vi "FPGA 796xR - Backup20170922A.vi"() -> ()   [LabVIEW 2015]
uses:
  Controls/FPGA_Frame State.ctl
  <vilib>/Platform/TimedLoop/XDataNode/timing_clust.ctl
  <vilib>/Platform/TimedLoop/XDataNode/nitl_modes.ctl
  <vilib>/Platform/TimedLoop/XDataNode/wakeup.ctl
  <vilib>/rvi/Emulation/niFpgaSctlEmulationGetInTimedLoop.vi
  <vilib>/rvi/Emulation/niFpgaProcessEmulError.vi
  <vilib>/rvi/Emulation/niFpgaEmulationReportErrorSimple.vi
  <vilib>/rvi/Emulation/niFpgaGetClockAttributes.vi
  <vilib>/rvi/Emulation/niFpgaCriticalErrorInLSC.vi
  <vilib>/rvi/eio/common/nirviEmuTemplateMethod_errors.vi
  <vilib>/rvi/Memory/Memory_Emulation/nirvimemoryFastEmulation.vi
  <vilib>/rvi/Memory/Memory_Emulation/nirvimemoryEmulation.vi
  <vilib>/rvi/Emulation/niFpgaEmulationIsFPGAContextNoSignature.vi
  <vilib>/rvi/DataTransferAndStorage/Container/Common/niFpgaContainerGetUniqueNameForEmu.vi
  <vilib>/rvi/errors/nirviReportUnexpectedCaseInternalError (U32).vi
  <vilib>/rvi/interface/RandomDataEmulation/niFpgaRandomDataHandleErrors.vi
  <vilib>/Platform/TimedLoop/XDataNode/XDataNode.xnode
  <vilib>/eio/EIONode/EIONode.xnode
  <vilib>/rvi/DataTransferAndStorage/Container/XNode/niFpgaContainer.xnode
  <vilib>/rvi/FXPMathLib/FxpMul/XNode/nifxpmath_Multiplier.xnode
  <vilib>/rvi/FXPMathLib/FxpAdd/XNode/nifxpmath_Add.xnode
  <vilib>/rvi/interface/RandomDataEmulation/nirviRandomDataFpgaReadWriteTemplate.vi
  <vilib>/Platform/TimedLoop/XDataNode/XDNodeRunTimeDep.lvlib
  <instrlib>/_niInstr/Basic Elements/v1/FPGA/niInstr Basic Elements v1 FPGA.lvlib
  <vilib>/rvi/FXPMathLib/sim/FxpSim.dll
panel:
  in  "Divide":u8
  out "Acq. Point Dis.":u16
  in  "Acq.Start":u16
  in  "Acq.Start FXP":fxp<+,18,0>
  out "Acq Pixel Number":u32
  out "AcqPoint 元素数量":u32
  in  "Microscope":enum16{"Miniature", "Benchtop"}(ring)
  in  "FOCUS":bool
  out "Wait Frame State":T1
  in  "Line":u16
  in  "Pixel/Line":u16
  out "Adapter Module Present":bool
  out "Adapter Module ID Expected":u32
  out "Adapter Module ID Inserted":u32
  out "Adapter Module Initialization Done":bool
  out "Adapter Module ID Mismatch":bool
  in  "Adapter Module Do User Command Commit":bool caption="(Mech Action: Latch)"
  in  "Adapter Module User Command":u8
  out "Adapter Module User Command Idle":bool
  out "Adapter Module User Command Status":u8
  in  "Adapter Module User Data 0":u8
  in  "Adapter Module User Data 1":u8
  out "Adapter Module PLL Locked":bool
  # "Acquisition Parameters"
  # "Acquisition Control"
  # "User Command Load"
  # "Fpga status"
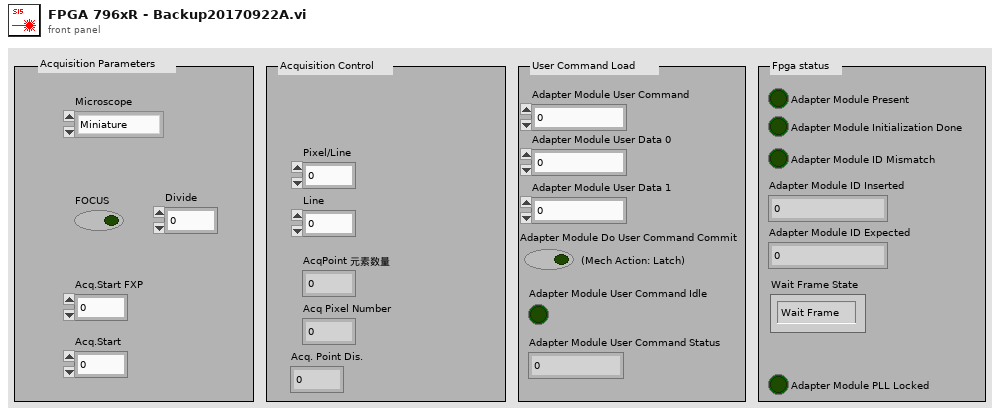
[diagram p1: front panel]
types:
  T1 = typedef "FPGA_Frame State.ctl" = enum16{"Wait Frame", "Start Frame", "Framing"}
  T2 = typedef "XDNodeRunTimeDep.lvlib/timing_clust.ctl" = cluster{"Expected End [f-1]":u64, "Actual End [f-1]":u64, "Finished Late? [f-1]":bool, "Expected End [i-1]":u64, "Actual End [i-1]":u64, "Finished Late? [i-1]":bool, "Expected Start [i]":u64, "Actual Start [i]":u64, "Expected Start [f]":u64, "Actual Start [f]":u64, "Source Name":string, "Structure Name":string, "Period":i64, "Deadline":i64, "Offset":i64, "Start":i64, "Priority":i32, "Timeout":i32, "Mode":T3, "Wakeup Reason":T4, "Error":errorcluster, "Source Type":string, "Secondary Source Type":string, "Global End Time":u64, "Global Start Time":u64, "Frame Duration":u64, "Iteration Duration":u64, "Assigned CPU":i32, "I/O Scan Engine Mode":u32}
  T3 = typedef "XDNodeRunTimeDep.lvlib/nitl_modes.ctl" = enum32{"No Change", "Process missed periods, maintain original phase", "Discard missed periods, maintain original phase", "Process missed periods, ignore original phase", "Discard missed periods, ignore original phase"}
  T4 = typedef "XDNodeRunTimeDep.lvlib/wakeup.ctl" = enum32{"Normal", "Aborted", "Asynchronous wakeup", "Timing source error", "Timed loop error", "Timeout"}
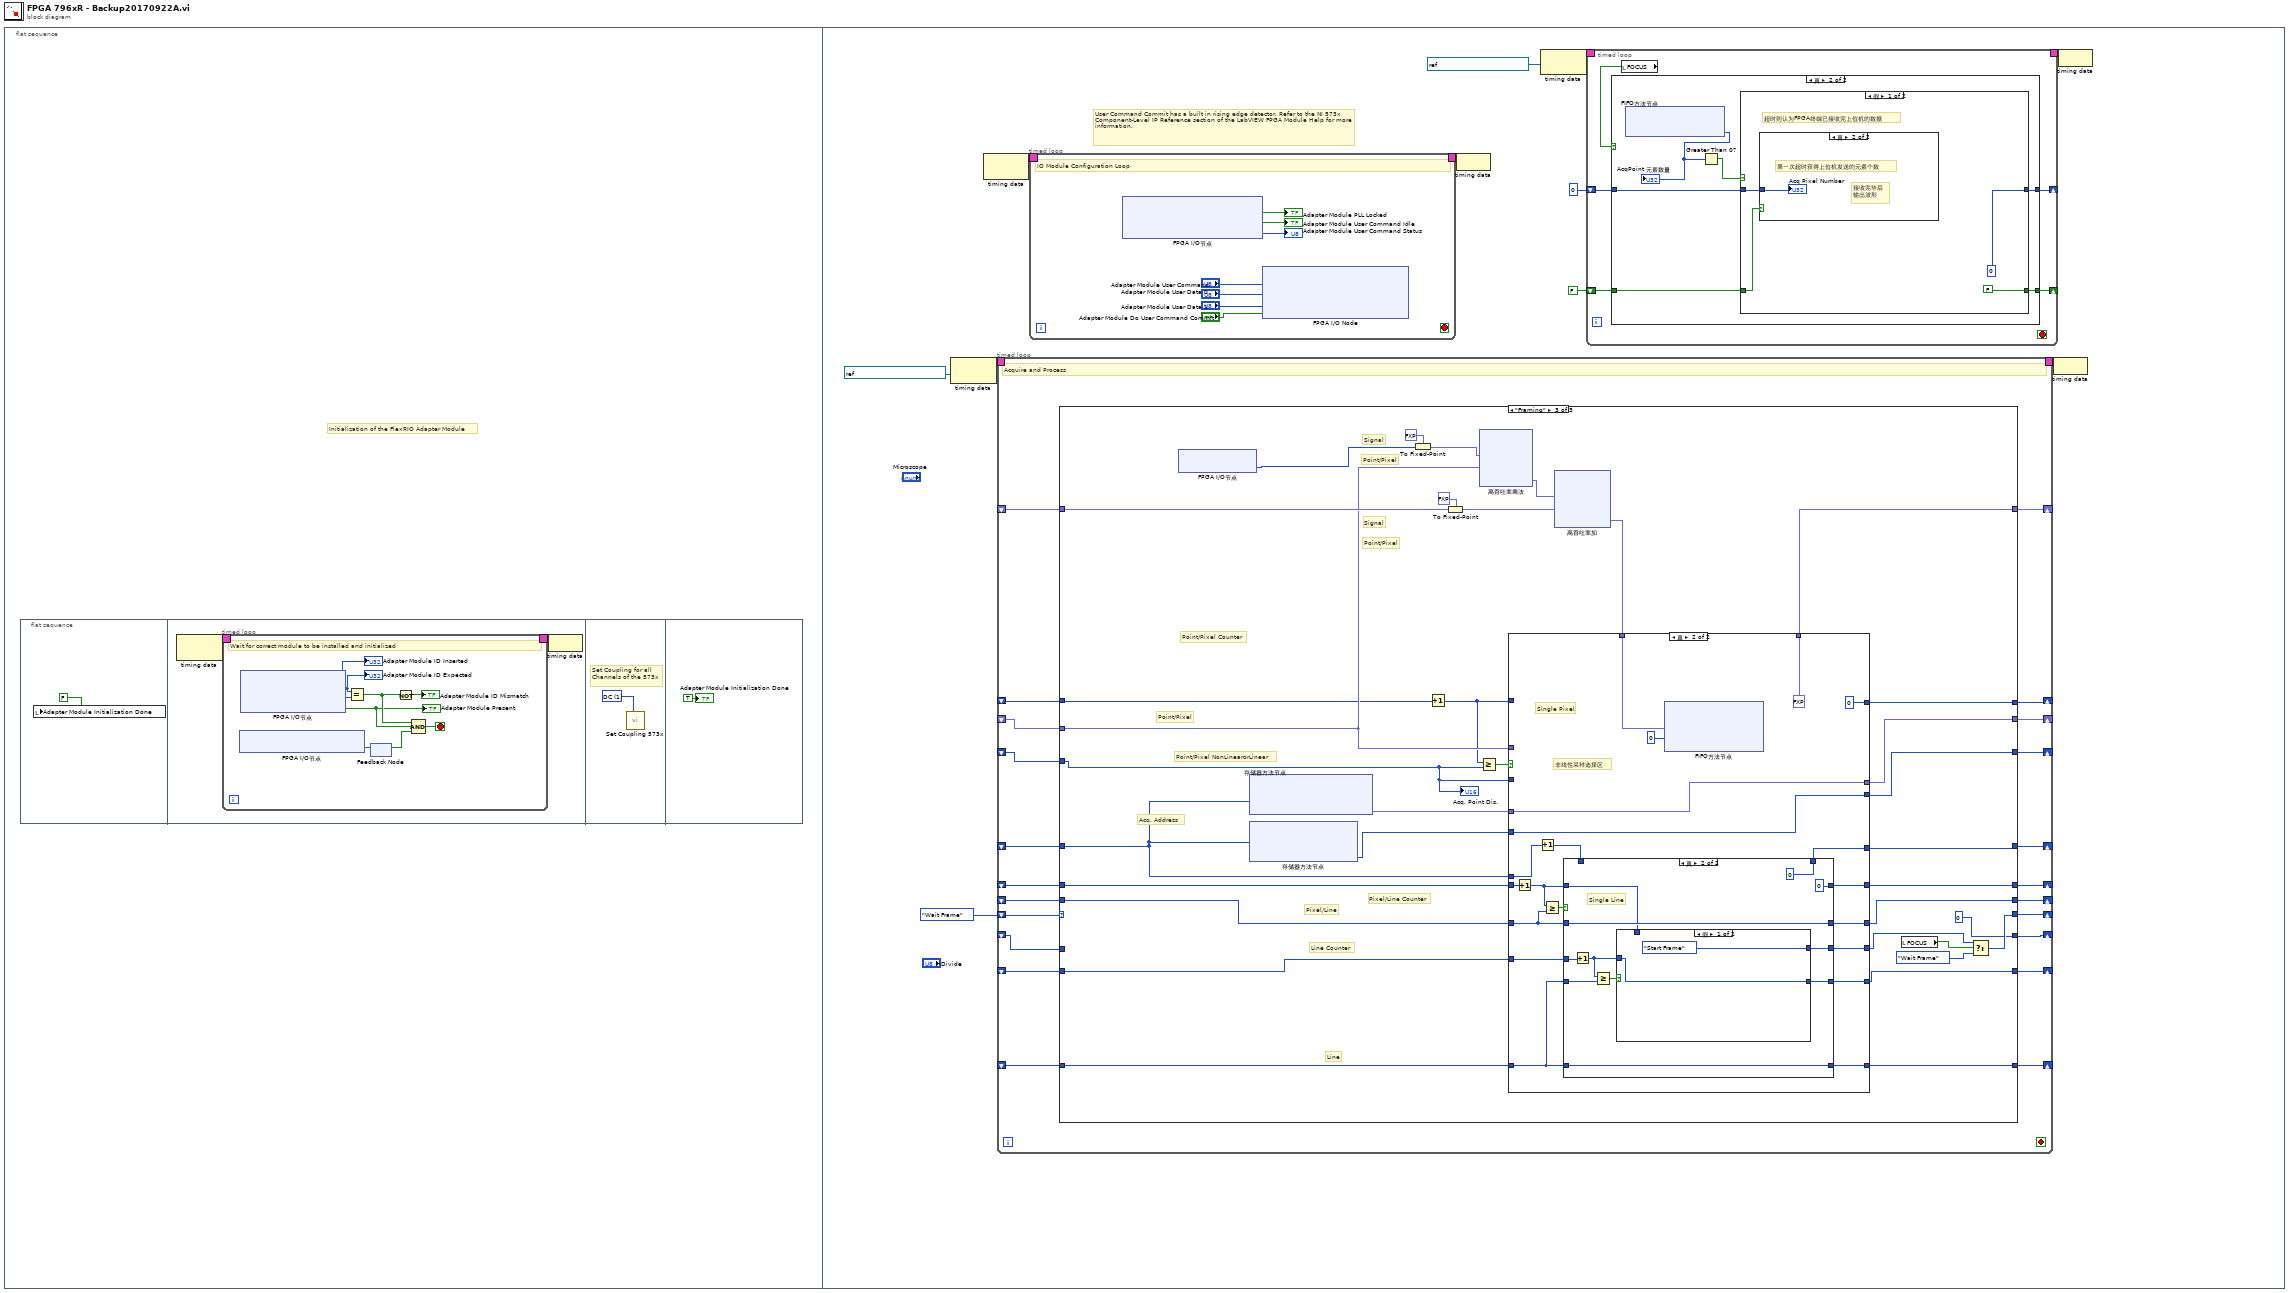
[diagram p0: block diagram]
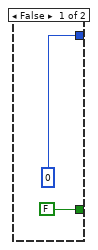
[diagram p2: hidden frame]
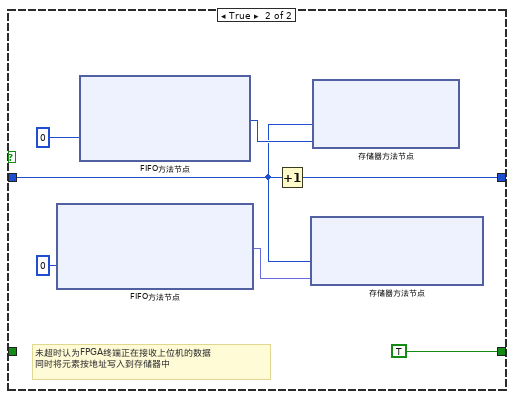
[diagram p4: hidden frame]
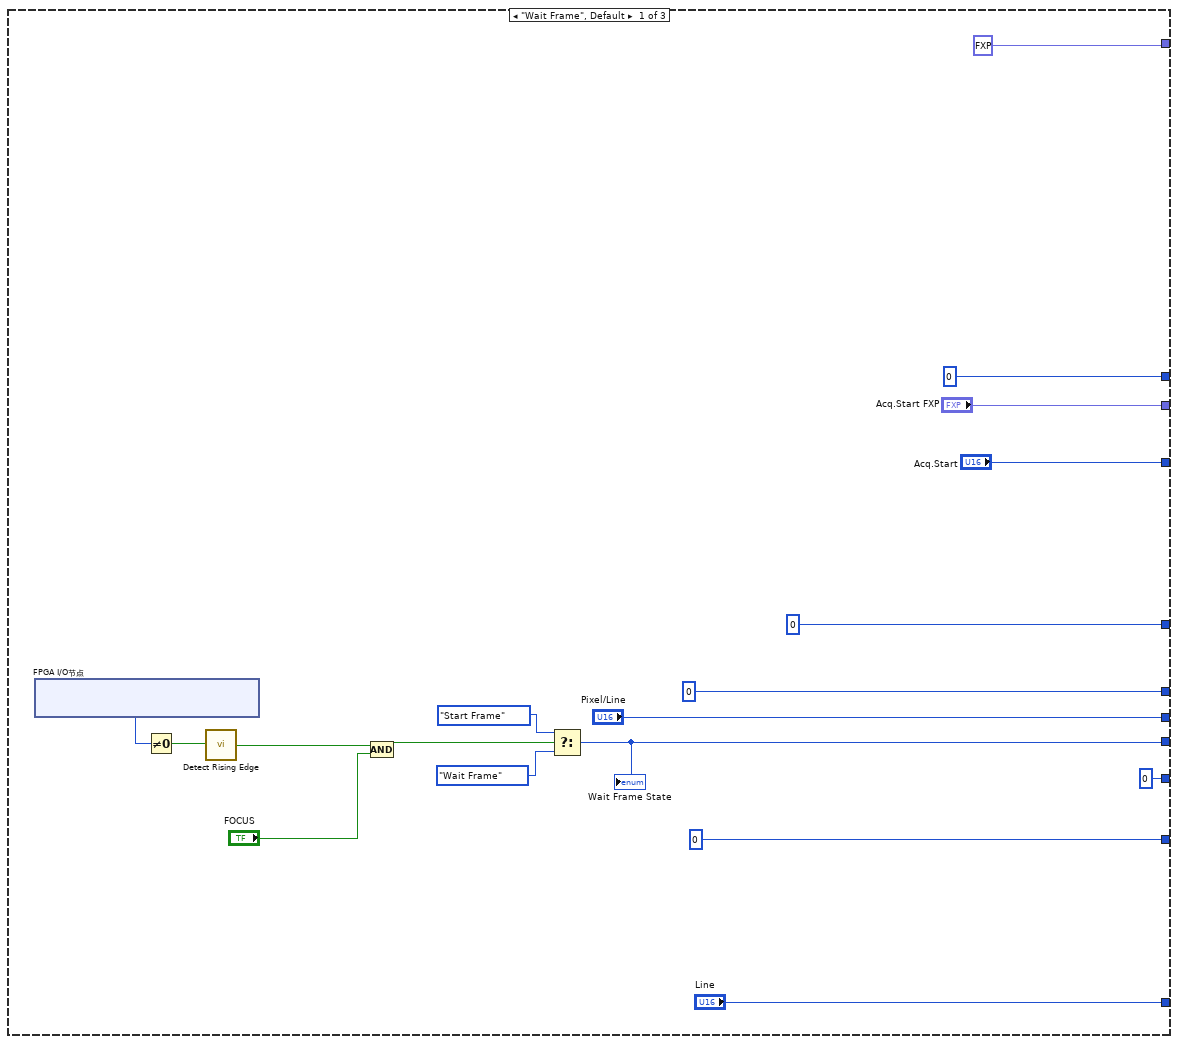
[diagram p5: hidden frame]
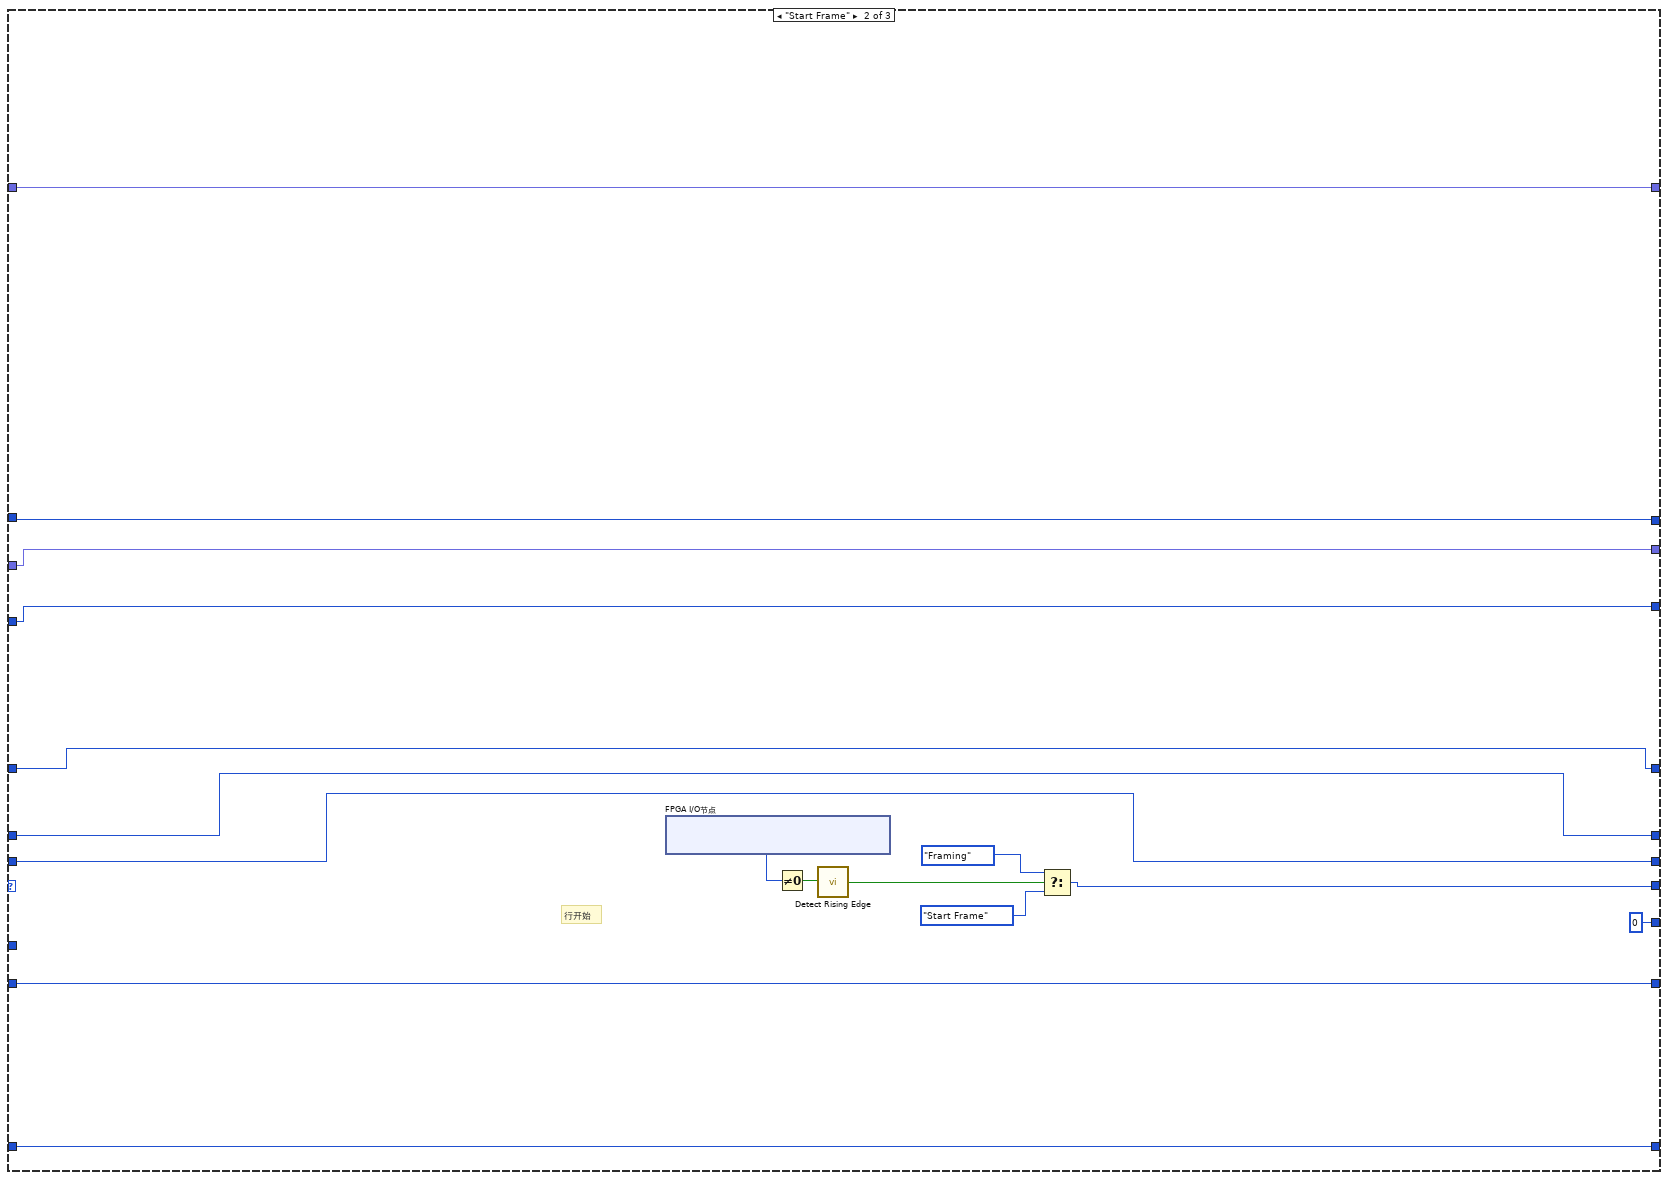
[diagram p6: hidden frame]
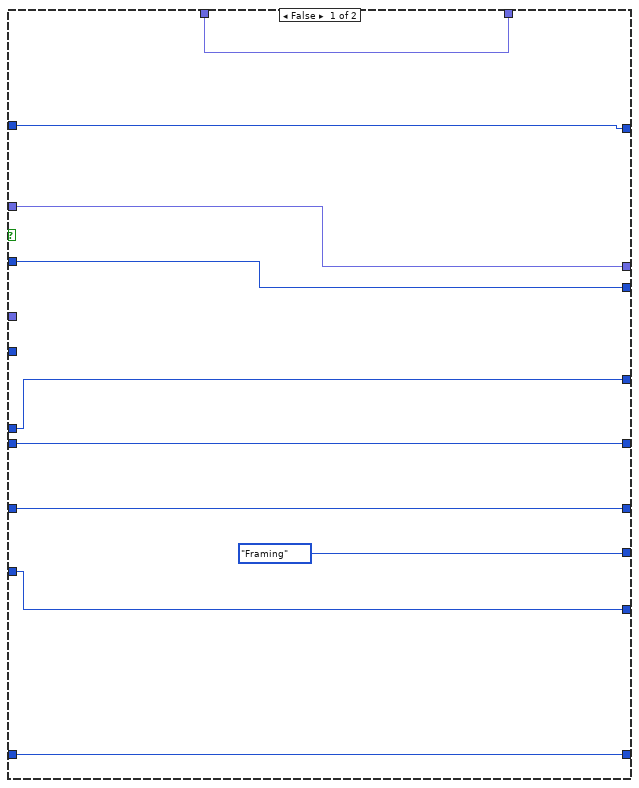
[diagram p7: hidden frame]
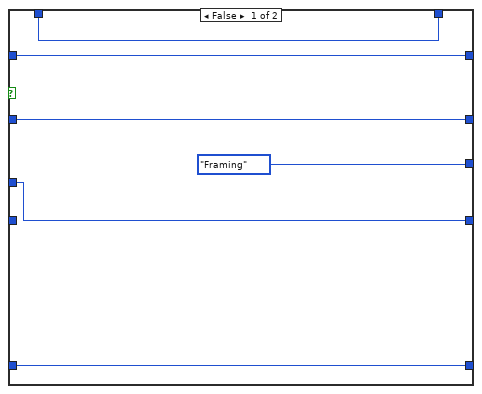
[diagram p8: hidden frame]
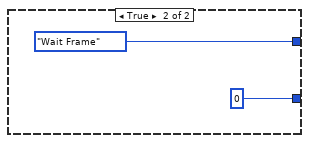
[diagram p9: hidden frame]
diagram:
  n1 = flat-sequence {
    frame #0 {
      # "Initialization of the FlexRIO Adapter Module"
      n2 = flat-sequence {
        frame #0 {
          n3 = local write "Adapter Module Initialization Done"(FALSE ("InitializationDone")) -> ()
        }
        frame #1 {
          n4 = node-c288() -> (w3:T2)  [unwired: 1 in]
          n5 = timed-loop {
            timing: w3 -> [_]
            timing-out: [_] -> w2
            stop <- w10 stop-if-true
            # "Wait for correct module to be installed and initialized"
            n6 = xnode "FPGA I/O节点"() -> ("IO Module\\Initialization Done"=w5:bool)  [unwired: 1 in, 1 out]
            n7 = xnode "FPGA I/O节点"() -> ("Expected IO Module ID"=w11:u32, "Inserted IO Module ID"=w9:u32, "IO Module Present"=w6:bool)  [unwired: 3 in, 3 out]
            "Adapter Module ID Inserted" <- w9
            "Adapter Module ID Expected" <- w11
            "Adapter Module Present" <- w6
            n8 = Equal?(x=w11, y=w9) -> (x = y?=w7:bool)
            n9 = feedback-in #1(w5) -> ()
            n10 = feedback #1() -> (w4:bool)  [unwired: 1 in]
            n11 = Not(x=w7) -> (.not. x?=→"Adapter Module ID Mismatch":bool)
            n12 = Compound Arithmetic op=AND(w7, w6, w4) -> (w10:bool)
          }
          n13 = node-c288(w2) -> ()
        }
        frame #2 {
          w16 = u8 1 items=["DC"=1, "AC"=0] ("Coupling")
          # "Set Coupling for all\nChannels of the 573x"
          n14 = call "Set Coupling 573x.vi"("Coupling"=w16) -> ()  [unwired: 11 in]
        }
        frame #3 {
          "Adapter Module Initialization Done" <- TRUE ("InitializationDone")
        }
      }
    }
    frame #1 {
      # "User Command Commit has a built in rising edge detector. Refer to the NI 573x Component-Level IP Reference section of the LabVIEW FPGA Module Help for more information."
      n15 = node-c288(refnum<k21> "IO Module\\Sample Clock" ("Source Name")) -> (w26:T2)
      n16 = node-c288() -> (w28:T2)  [unwired: 1 in]
      n17 = timed-loop {
        timing: w26 -> [_]
        timing-out: [_] -> w25
        shift-right: [w80] -> _
        shift-left: FPGA_Frame_State."Wait Frame" ("Line State") -> [w81]
        shift-right: [w78] -> _
        shift-left: _ -> [w79]
        shift-right: [w76] -> _
        shift-left: _ -> [w77]
        shift-right: [w74] -> _
        shift-left: _ -> [w75]
        shift-right: [w72] -> _
        shift-left: _ -> [w73]
        shift-right: [w70] -> _
        shift-left: _ -> [w71]
        shift-right: [w68] -> _
        shift-left: _ -> [w69]
        shift-right: [w66] -> _
        shift-left: _ -> [w67]
        shift-right: [w64] -> _
        shift-left: _ -> [w65]
        shift-right: [w63] -> _
        shift-left: _ -> [w62]
        shift-right: [w60] -> _
        shift-left: _ -> [w61]
        stop <- _ stop-if-true
        # "Acquire and Process"
        n18 = case shown="\"Framing\"" w81 {
          tunnel: [w95 w111 w149] -> w80
          tunnel: w79 -> [_ w103 w131]
          tunnel: [u16 0 ("t") w103 w148] -> w78
          tunnel: w77 -> [_ w105 w147]
          tunnel: [u16 0 ("t") w105 w146] -> w76
          tunnel: w75 -> [_ w104 w145]
          tunnel: [fxp<+,32,16> 0.0 ("x") w104 w144] -> w74
          tunnel: w73 -> [_ w113 w143]
          tunnel: [u16 0 ("t") w113 w142] -> w72
          tunnel: w71 -> [_ w108 w134]
          tunnel: ["Acq.Start FXP" w108 w137] -> w70
          tunnel: w69 -> [_ w107 w141]
          tunnel: ["Pixel/Line" w107 w140] -> w68
          tunnel: w67 -> [_ w106 w139]
          tunnel: ["Line" w106 w138] -> w66
          tunnel: w65 -> [_ w102 w132]
          tunnel: ["Acq.Start" w102 w136] -> w64
          tunnel: [u32 0 ("地址") w101 w135] -> w63
          tunnel: w62 -> [_ w101 w133]
          tunnel: w61 -> [_ _ _]
          tunnel: [u8 0 u8 0 u8 0] -> w60
          frame "Wait Frame", Default {
            n19 = xnode "FPGA I/O节点"() -> ("IO Module\\DIO Port 1 Rd Data"=w97:u8)  [unwired: 1 in, 1 out]
            n20 = Not Equal To 0?(x=w97) -> (x != 0?=w98:bool)
            n21 = call <instrlib>:"Detect Rising Edge.vi"("signal"=w98) -> ("edge detected"=w87:bool)  [unwired: 14 in]
            n22 = Compound Arithmetic op=AND(w87, "FOCUS") -> (w88:bool)
            n23 = Select(t=FPGA_Frame_State."Start Frame" ("Line State"), s=w88, f=FPGA_Frame_State."Wait Frame" ("Line State")) -> (s? t:f=w95:T1)
            "Wait Frame State" <- w95
          }
          frame "Start Frame" {
            # "行开始"
            n24 = xnode "FPGA I/O节点"() -> ("IO Module\\DIO Port 0 Rd Data"=w114:u8)  [unwired: 1 in, 1 out]
            n25 = Not Equal To 0?(x=w114) -> (x != 0?=w115:bool)
            n26 = call <instrlib>:"Detect Rising Edge.vi"("signal"=w115) -> ("edge detected"=w112:bool)  [unwired: 14 in]
            n27 = Select(t=FPGA_Frame_State."Framing" ("Line State"), s=w112, f=FPGA_Frame_State."Start Frame" ("Line State")) -> (s? t:f=w111:T1)
          }
          frame "Framing" {
            # "Acq. Address"
            # "Pixel/Line Counter"
            # "Point/Pixel NonLinearorLinear"
            # "Signal"
            # "Signal"
            # "Point/Pixel"
            # "Point/Pixel"
            # "Line Counter"
            # "Line"
            # "Point/Pixel Counter"
            # "Pixel/Line"
            # "Point/Pixel"
            n28 = xnode "FPGA I/O节点"() -> ("IO Module\\AI 1"=w119:u16)  [unwired: 1 in, 1 out]
            n29 = xnode ("存储器方法节点")("地址"=w133) -> ("数据"=w121:fxp<+,18,0>)  [unwired: 1 in, 1 out]
            n30 = xnode ("存储器方法节点")("地址"=w133) -> ("数据"=w122:u16)  [unwired: 1 in, 1 out]
            n31 = To Fixed-Point(fixed-point type=fxp<+,16,16> 0.0 ("x"), number=w119) -> (fixed-point=w123:fxp<+,16,16>)
            n32 = Increment(x=w131) -> (x+1=w120:u16)
            n33 = To Fixed-Point(fixed-point type=fxp<+,32,16> 0.0 ("x"), number=w145) -> (fixed-point=w117:fxp<+,32,16>)
            n34 = xnode ("高吞吐率乘法")("x"=w123, "y"=w134) -> ("x*y"=w118:fxp<+,32,16>)
            n35 = Greater Or Equal?(x=w120, y=w132) -> (x >= y?=w127:bool)
            n36 = xnode ("高吞吐率加")("x"=w118, "y"=w117) -> ("x+y"=w116:fxp<+,33,17>)
            n37 = case shown="真" w127 {
              tunnel: w116 -> [w151 w165]
              tunnel: [w151 fxp<+,32,16> 0.0 ("x")] -> w144
              tunnel: [w150 u16 0 ("t")] -> w148
              tunnel: w120 -> [w150 _]
              tunnel: w147 -> [w156 w171]
              tunnel: w143 -> [w155 w177]
              tunnel: [w155 w176] -> w142
              tunnel: [FPGA_Frame_State."Framing" ("Line State") w175] -> w125
              tunnel: [w156 w170] -> w146
              tunnel: w139 -> [w158 w173]
              tunnel: [w157 w172] -> w140
              tunnel: w141 -> [w157 w167]
              tunnel: [w158 w174] -> w138
              tunnel: w134 -> [w154 _]
              tunnel: [w154 w162] -> w137
              tunnel: w132 -> [w153 _]
              tunnel: [w153 w161] -> w136
              tunnel: w122 -> [_ w161]
              tunnel: [w152 w163] -> w135
              tunnel: w121 -> [_ w162]
              tunnel: w133 -> [w152 w160]
              frame False {
              }
              frame True {
                # "Single Pixel"
                # "非线性采样选择区"
                n38 = Increment(x=w171) -> (x+1=w166:u16)
                n39 = Increment(x=w160) -> (x+1=w164:u32)
                n40 = Greater Or Equal?(x=w166, y=w167) -> (x >= y?=w169:bool)
                n41 = case shown="真" w169 {
                  tunnel: w177 -> [w181 w196]
                  tunnel: [w181 w195] -> w176
                  tunnel: [FPGA_Frame_State."Framing" ("Line State") w194] -> w175
                  tunnel: w173 -> [_ w191]
                  tunnel: [w185 w190] -> w174
                  tunnel: w173 -> [w185 w190]
                  tunnel: [w184 w189] -> w172
                  tunnel: w167 -> [w184 w189]
                  tunnel: [w183 u16 0] -> w170
                  tunnel: w166 -> [w183 w187]
                  tunnel: w164 -> [w180 _]
                  tunnel: [w180 u32 0] -> w163
                  frame False {
                  }
                  frame True {
                    # "Single Line"
                    n42 = Increment(x=w196) -> (x+1=w192:u16)
                    n43 = Greater Or Equal?(x=w192, y=w191) -> (x >= y?=w193:bool)
                    n44 = case shown="假" w193 {
                      tunnel: w192 -> [w197 _]
                      tunnel: [w197 u16 0] -> w195
                      tunnel: [FPGA_Frame_State."Start Frame" ("Line State") FPGA_Frame_State."Wait Frame" ("Line State")] -> w194
                      tunnel: w187 -> [_ _]
                      frame False {
                      }
                      frame True {
                      }
                    }
                  }
                }
                n45 = xnode ("FIFO方法节点")("元素"=w165, "超时"=0) -> ()  [unwired: 1 in, 2 out]
              }
            }
            n46 = local read "FOCUS"() -> (w126:bool)
            n47 = Select(t=w125, s=w126, f=FPGA_Frame_State."Wait Frame" ("Line State")) -> (s? t:f=w149:T1)
            "Acq. Point Dis." <- w132
          }
        }
      }
      n48 = timed-loop {
        timing: w28 -> [_]
        timing-out: [_] -> w27
        stop <- _ stop-if-true
        # "IO Module Configuration Loop"
        n49 = xnode "FPGA I/O节点"() -> ("IO Module\\PLL Locked"=→"Adapter Module PLL Locked":bool, "IO Module\\User Command Idle"=→"Adapter Module User Command Idle":bool, "IO Module\\User Command Status"=→"Adapter Module User Command Status":u8)  [unwired: 3 in, 3 out]
        n50 = xnode ("FPGA I/O Node")("IO Module\\User Command"="Adapter Module User Command", "IO Module\\User Data 0"="Adapter Module User Data 0", "IO Module\\User Data 1"="Adapter Module User Data 1", "IO Module\\User Command Commit"="Adapter Module Do User Command Commit") -> ()  [unwired: 4 in, 4 out]
      }
      n51 = node-c288(w27) -> ()
      n52 = node-c288(refnum<k21> "IO Module\\Sample Clock" ("Source Name")) -> (w22:T2)
      n53 = timed-loop {
        shift-right: [w32] -> _
        shift-left: u32 0 ("地址") -> [w33]
        shift-right: [w30] -> _
        shift-left: FALSE ("执行") -> [w31]
        timing: w22 -> [_]
        timing-out: [_] -> w21
        stop <- _ stop-if-true
        n54 = local read "FOCUS"() -> (w29:bool)
        n55 = case shown="真" w29 {
          tunnel: w33 -> [_ w41]
          tunnel: [u32 0 w40] -> w32
          tunnel: w31 -> [_ w39]
          tunnel: [FALSE w38] -> w30
          frame False {
          }
          frame True {
            n56 = xnode ("FIFO方法节点")() -> ("待读取元素数量"=w36:u32)  [unwired: 1 in, 1 out]
            "AcqPoint 元素数量" <- w36
            n57 = Greater Than 0?(x=w36) -> (x > 0?=w37:bool)
            n58 = case shown="假" w37 {
              tunnel: w41 -> [w43 w47]
              tunnel: [u32 0 w52] -> w40
              tunnel: w39 -> [w44 _]
              tunnel: [FALSE TRUE] -> w38
              frame False {
                # "超时则认为FPGA终端已接收完上位机的数据"
                n59 = case shown="真" w44 {
                  tunnel: w43 -> [_ w46]
                  frame False {
                  }
                  frame True {
                    # "接收完毕后\n输出波形"
                    # "第一次超时获得上位机发送的元素个数"
                    "Acq Pixel Number" <- w46
                  }
                }
              }
              frame True {
                # "未超时认为FPGA终端正在接收上位机的数据\n同时将元素按地址写入到存储器中"
                n60 = xnode ("FIFO方法节点")("超时"=0) -> ("元素"=w49:fxp<+,18,0>)  [unwired: 1 in, 2 out]
                n61 = xnode ("FIFO方法节点")("超时"=0) -> ("元素"=w50:u16)  [unwired: 1 in, 2 out]
                n62 = Increment(x=w47) -> (x+1=w52:u32)
                n63 = xnode ("存储器方法节点")("地址"=w47, "数据"=w49) -> ()  [unwired: 1 in, 1 out]
                n64 = xnode ("存储器方法节点")("地址"=w47, "数据"=w50) -> ()  [unwired: 1 in, 1 out]
              }
            }
          }
        }
      }
      n65 = node-c288(w25) -> ()
      n66 = node-c288(w21) -> ()
    }
  }
